vi "EnableCheck.vi"(1 "Enable?":bool) -> (0 "Enum":T1(ring))   [LabVIEW 2020]
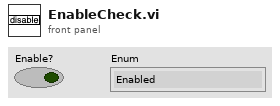
[diagram p1: front panel]
types:
  T1 = enum8{"Enabled", "Disabled", "Disabled and Grayed Out"}
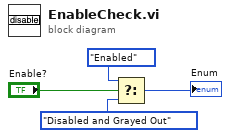
[diagram p0: block diagram]
diagram:
  n1 = Select(t=T1."Enabled" ("Disabled"), s="Enable?", f=T1."Disabled and Grayed Out" ("Disabled")) -> (s? t:f=→"Enum":T1)
